vi "Digitizer Scan Fetch FFT Magnitude.vi"(0 "instrument handle":refnum<k15>, 1 "Length":i32 format="%.0g", 2 "ValBufferSize":i32=2048, 5 "Function (Flat)":i32(ring) items=["Flat", "Hanning"], 7 "Record":i32 format="%.0g", 9 "FirstPoint":i32 format="%.0g", 11 "error in (no error)":errorcluster {"code" format="%.0x"}, 12 "Channel":string) -> (4 "instrument handle out":refnum<k15>, 6 "Val":dbl[](array[numeric]) format="%.2p", 8 "ValActualSize":i32, 15 "error out":errorcluster {"code" format="%.0x"})   [LabVIEW 2020, in "Keysight DAQ970.lvlib"]
doc: "Performs post-processing calculation on the specified range of readings and returns FFT magnitude on the specified record for a channel."
uses:
  Keysight DAQ970.lvlib
  KtDAQ970.dll
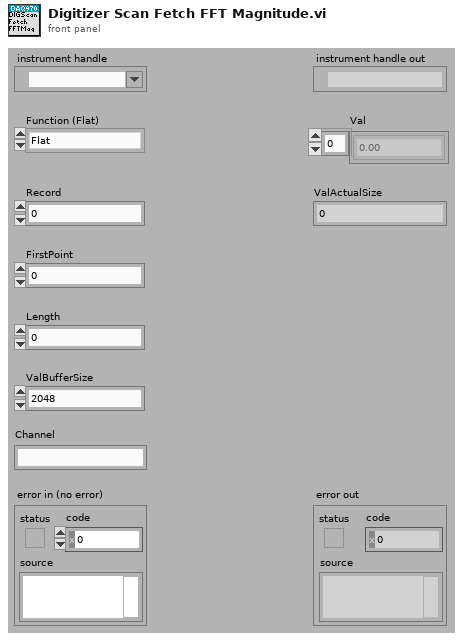
[diagram p1: front panel]
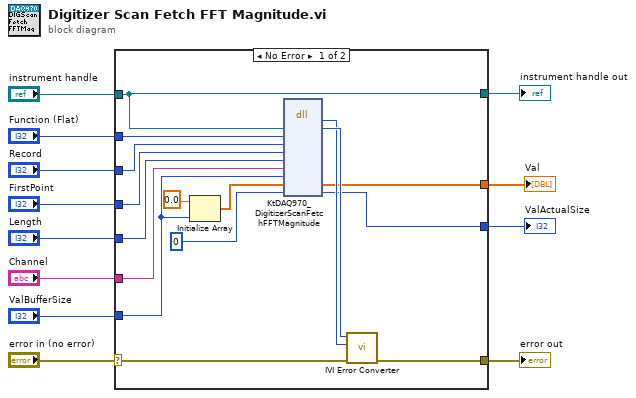
[diagram p0: block diagram]
diagram:
  n1 = case shown="No Error" "error in (no error)" {
    selector: "error in (no error)" -> [w26 w30]
    tunnel: [w25 w30] -> w12
    tunnel: "instrument handle" -> [w14 w29]
    tunnel: "Function (Flat)" -> [w24 _]
    tunnel: "Record" -> [w23 _]
    tunnel: "FirstPoint" -> [w22 _]
    tunnel: "Length" -> [w21 _]
    tunnel: "Channel" -> [w20 _]
    tunnel: "ValBufferSize" -> [w13 _]
    tunnel: [w17 _] -> w3
    tunnel: [w15 _] -> w2
    tunnel: [w14 w29] -> w1
    frame No Error {
      n2 = Initialize Array(0.0 ("element"), w13) -> (w19:dbl[])
      n3 = dll-call lib="KtDAQ970**.dll" fn="KtDAQ970_DigitizerScanFetchFFTMagnitude"("Vi"=w14, "Function"=w24, "Record"=w23, "FirstPoint"=w22, "Length"=w21, "Channel"=w20, "ValBufferSize"=w13, "Val"=w19, "ValActualSize"=0) -> (w27:i32, "Vi"=w28:u32, "Val"=w17:dbl[], "ValActualSize"=w15:i32)  [unwired: 9 in, 2 out]
      n4 = call "IVI Error Converter.vi"("error in (no error)"=w26, "IVI error code (0)"=w27, "instrument handle"=w28) -> ("error out"=w25:errorcluster)  [unwired: 7 in, 1 out]
    }
    frame Error {
    }
  }
  "error out" <- w12
  "instrument handle out" <- w1
  "Val" <- w3
  "ValActualSize" <- w2
